vi "SPC_get_photons_from_stream.vi"(6 "Stream Handle":i16, 7 "EventCount":u32, 8 "Error In":errorcluster={"Status"=FALSE, "Code"=0, "Source"="\u0000\u0000\u0000\u0000\u0000\u0000\u0000\u0000\u0000\u0000\u0000\u0000\u0000\u0000\u0000\u0000\u0000\u0000\u0000\u0000\u0000\u0000\u0000\u0000\u0000\u0000\u0000\u0000\u0000\u0000\u0000\u0000\u0000\u0000\u0000\u0000\u0000\u0000\u0000\u0000\u0000\u0000\u0000\u0000\u0000\u0000\u0000\u0000\u0000\u0000\u0000\u0000\u0000\u0000\u0000\u0000\u0000\u0000\u0000\u0000\u0000\u0000\u0000\u0000"}, 10 "Module No":i16=2, 11 "DLL Path":path=path "C:/Program Files (x86)/BH/SPCM/DLL/spcm64.dll") -> (0 "Error Out":errorcluster, 1 "phot_no":i32, 2 "Module No":i16=2, 3 "DLL Path":path=path "C:/Program Files (x86)/BH/SPCM/DLL/spcm64.dll", 4 "Stream Handle":i16, 5 "PhotInfo64":T1[](array[typedef]) {"flags" max=3 format="%016b"; "rout_chan" step=1; "micro_time" step=1; "mtime" step=1})   [LabVIEW 2017]
doc: "EventCount: contains required number of photons to extract from buffered stream ‘stream_hndl’, 1 .. 1000000\nphot_no: number of photons extracted from buffered stream ‘stream_hndl’\nReturn value (Error Out): >= 0: no errors, 1 – stop condition found, 2 – end of the stream reached <0: error code\nThe procedure is used to extract photons data from the opened 'buffered' photons streamdefined by handle 'stream_hndl'. \nPhotons data are packed to the structures PhotInfo64 (defined in spcm_def.h file) in 'phot_info' buffer.\nEventCount is the upper limit number of expected photons; used for array allocation. EventCount is limited by the dll to 1000000.\nThe 'phot_no' variable is filled on exit with the number of photons actually extracted from the stream.\nExtracting photons can be done also during running measurement. During extracting or adding photons the stream is locked. Only one thread can access the thread safe stream at a time. If a thread requests the access to stream resources while another has it, the second thread waits in this function until the first thread releases the stream.\nUsing SPC_stream_start_condition and SPC_stream_stop_condition user can define start/stop condition of extracting photons, which can be specific macro time and/or occurrence of markers or routing channels.\nUser can define start and stop condition for extracting photons using functions SPC_stream_start(stop)_condition. \nThe condition can be a specified macro time value and/or occurrence of specific markers and/or routing channels. See description of SPC_stream_start(stop)_condition functions.\nPhotons extracted to 'phot_info' buffer can be saved to .ph file.\nFirst 4 bytes of .ph file it is a header ( the same as for .spc files). Call SPC_get_fifo_init_vars to get the header value. After the header subsequent PhotInfo64 photons structures are stored. \nSuch file can be used in SPCM software as an input file in 'Convert FIFO Files' panel. \n\ninfo@becker-hickl.com"
uses:
  SPC_Controls/SPC_PhotInfo64.ctl
panel:
  out "phot_info":u8[](array[numeric])
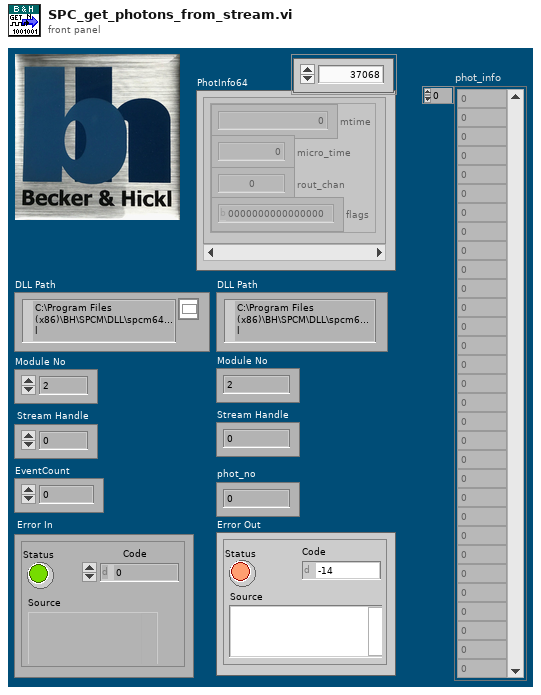
[diagram p1: front panel]
types:
  T1 = typedef "SPC_PhotInfo64.ctl" = cluster{"mtime":u64, "micro_time":u16, "rout_chan":u16, "flags":u16}
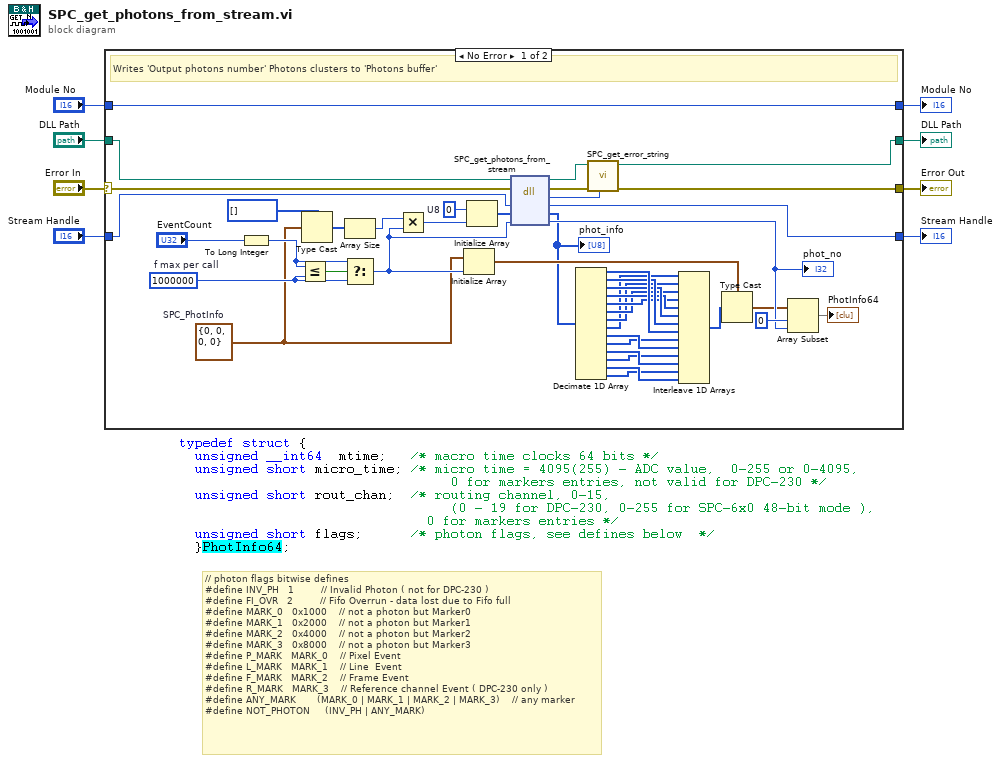
[diagram p0: block diagram]
diagram:
  # "// photon flags bitwise defines\n#define INV_PH   1         // Invalid Photon ( not for DPC-230 )    \n#define FI_OVR   2         // Fifo Overrun - data lost due to Fifo full\n#define MARK_0   0x1000    // not a photon but Marker0\n#define MARK_1   0x2000    // not a photon but Marker1\n#define MARK_2   0x4000    // not a photon but Marker2\n#define MARK_3   0x8000    // not a photon but Marker3\n#define P_MARK   MARK_0    // Pixel Event \n#define L_MARK   MARK_1    // Line  Event \n#define F_MARK   MARK_2    // Frame Event \n#define R_MARK   MARK_3    // Reference channel Event ( DPC-230 only )\n#define ANY_MARK       (MARK_0 | MARK_1 | MARK_2 | MARK_3)    // any marker\n#define NOT_PHOTON     (INV_PH | ANY_MARK)"
  n1 = case shown="No Error" "Error In" {
    selector: "Error In" -> [w49 w55]
    tunnel: "DLL Path" -> [w48 w54]
    tunnel: [w45 w54] -> w6
    tunnel: [w39 w55] -> w5
    tunnel: [w38 w53] -> w4
    tunnel: "Stream Handle" -> [w43 w53]
    tunnel: "Module No" -> [w42 w52]
    tunnel: [w42 w52] -> w1
    frame No Error {
      w30 = T1 {"mtime"=0, "micro_time"=0, "rout_chan"=0, "flags"=0}  # SPC_PhotInfo
      w37 = u8 0  # U8
      w51 = 1000000  # f max per call
      # "Writes 'Output photons number' Photons clusters to 'Photons buffer'"
      n2 = To Long Integer(number="EventCount") -> (32bit integer=w40:i32)
      n3 = Less Or Equal?(x=w40, y=w51) -> (x <= y?=w50:bool)
      n4 = Type Cast(type=u8[] [], x=w30) -> (*(type *) &x=w35:u8[])
      n5 = Array Size(array=w35) -> (size(s)=w28:i32)
      n6 = Select(t=w40, s=w50, f=w51) -> (s? t:f=w33:i32)
      n7 = Multiply(x=w28, y=w33) -> (x*y=w32:i32)
      n8 = Initialize Array(w30, w33) -> (w26:T1[])
      n9 = Initialize Array(w37, w32) -> (w36:u8[])
      n10 = dll-call lib="C:/Program Files (x86)/BH/SPCM/DLL/spcm64.dll" fn="SPC_get_photons_from_stream"(path in=w48, error in=w49, "stream_hndl"=w43, "phot_info"=w36, "phot_no"=w33) -> (path out=w47:path, error out=w46:errorcluster, "return type"=w44:i16, "stream_hndl"=w38:i16, "phot_info"=w25:u8[], "phot_no"=w27:i32)  [unwired: 1 in]
      "phot_no" <- w27
      "phot_info" <- w25
      n11 = Decimate 1D Array(w25) -> (w23:u8[], w22:u8[], w21:u8[], w20:u8[], w19:u8[], w18:u8[], w17:u8[], w16:u8[], w15:u8[], w14:u8[], w13:u8[], w12:u8[], w11:u8[], w10:u8[])
      n12 = call "SPC_get_error_string.vi"("ErrorID"=w44, "Error In"=w46, "DLL Path"=w47) -> ("Error Out"=w39:errorcluster, "DLL Path"=w45:path)  [unwired: 6 in, 1 out]
      n13 = Interleave 1D Arrays(w16, w17, w18, w19, w20, w21, w22, w23, w14, w15, w12, w13, w10, w11) -> (w9:u8[])
      n14 = Type Cast(type=w26, x=w9) -> (*(type *) &x=w24:T1[])
      n15 = Array Subset(array=w24, index=0, length=w27) -> (→"PhotInfo64":T1[])
    }
    frame Error {
    }
  }
  "DLL Path" <- w6
  "Error Out" <- w5
  "Stream Handle" <- w4
  "Module No" <- w1
